vi "Step 7.vi"(8 "error in (no error)":errorcluster, 10 "Water Heater Type":T1, 11 "HeatUp Data in":string[][](array[string])) -> (0 "error out":errorcluster, 1 "110-130 Array":dbl[][](array[numeric]), 2 "Total Energy Expended (W-hr)":dbl, 3 "HP Recovery Time":dbl format="%#.4g", 4 "Watt Hours":cluster{"DBL":dbl[], "DBL":dbl[]}(graph), 5 "TC Avg":cluster{"DBL":dbl[], "DBL":dbl[]}(graph))   [LabVIEW 2016]
uses:
  Type Definitions/HEWH_Type.ctl
  Utility/Custom Pallet Controls/Custom Pallet String.ctl
  <vilib>/Utility/error.llb/DialogType.ctl
panel:
  out "Raw Data":string[][](array[string])
  # "Data with Stripped Header"
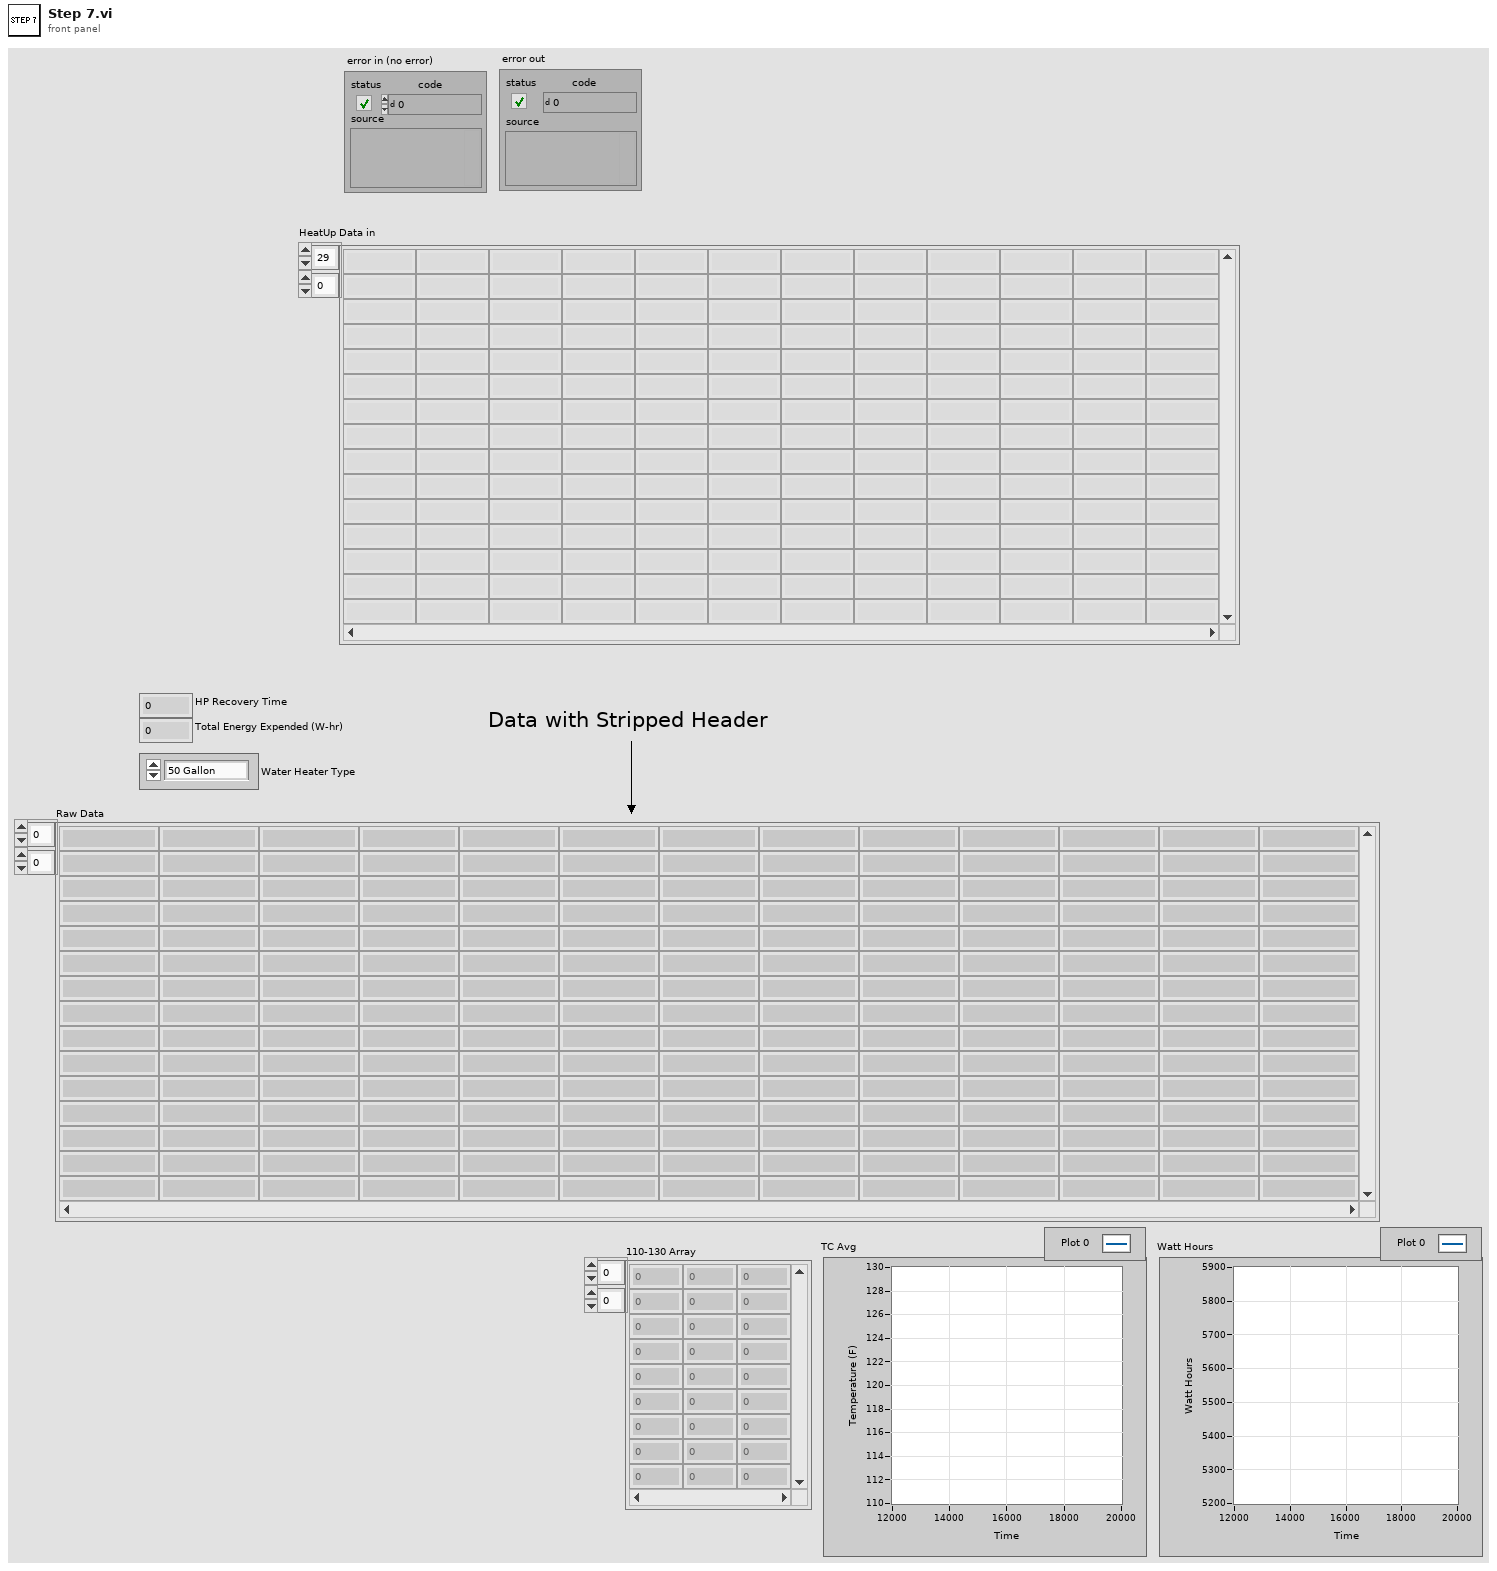
[diagram p1: front panel]
types:
  T1 = typedef "HEWH_Type.ctl" = enum16{"50 Gallon", "80 Gallon"}
  T2 = typedef "Custom Pallet String.ctl" = string
  T3 = cluster{"110-130 Array":dbl[], "110-130 Array":dbl[]}
  T4 = typedef "DialogType.ctl" = u16
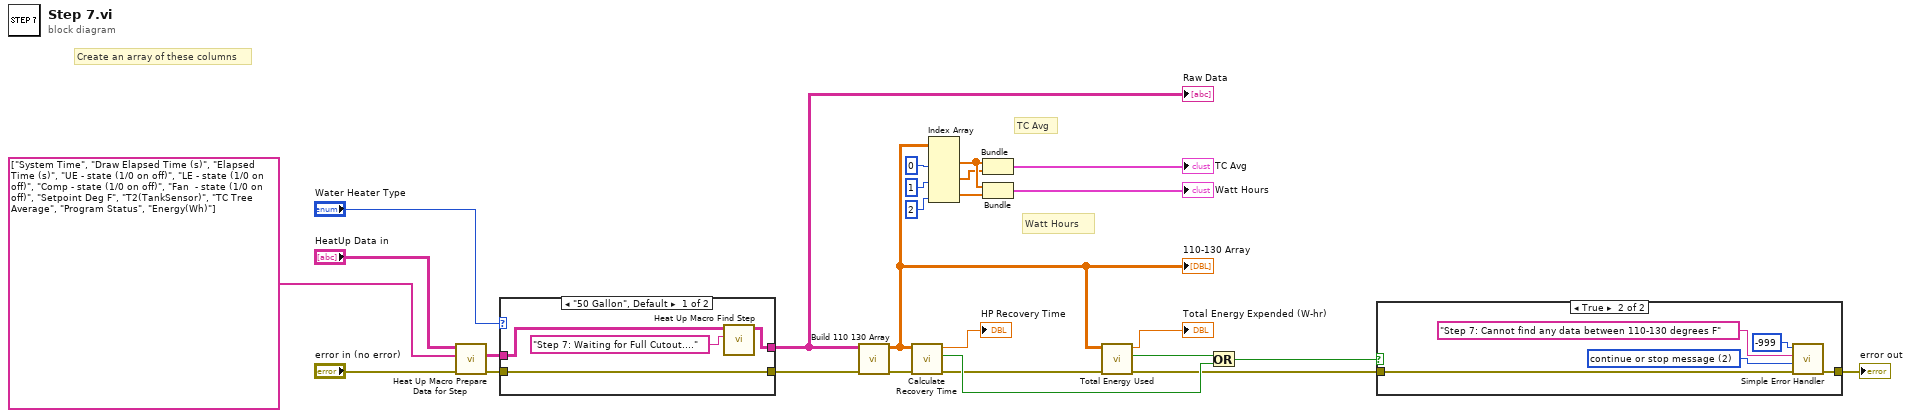
[diagram p0: block diagram]
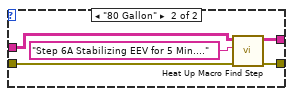
[diagram p2: hidden frame]
diagram:
  # "Watt Hours"
  # "TC Avg"
  # "Create an array of these columns"
  n1 = call "Heat Up Macro Prepare Data for Step.vi"("Error In"="error in (no error)", "Columns Too Search For"=string[] ["System Time", "Draw Elapsed Time (s)", "Elapsed Time (s)", "UE - state (1/0 on off)", "LE - state (1/0 on off)", "Comp - state (1/0 on off)", "Fan  - state (1/0 on off)", "Setpoint Deg F", "T2(TankSensor)", "TC Tree Average", "Program Status", "Energy(Wh)"], "HeatUp Raw Data Input"="HeatUp Data in") -> ("Error Out"=w6:errorcluster, "Heat Up Data with Only Selected Columns"=w9:string[][])  [unwired: 7 in]
  n2 = case shown="\"50 Gallon\", Default" "Water Heater Type" {
    tunnel: w9 -> [w30 w35]
    tunnel: [w28 w33] -> w8
    tunnel: w6 -> [w27 w32]
    tunnel: [w27 w31] -> w5
    frame "50 Gallon", Default {
      n3 = call "Heat Up Macro Find Step.vi"("Search For Step Name"=T2 "Step 7: Waiting for Full Cutout...." ("Message"), "Heat Up Data with Only Selected Columns"=w30) -> ("Filtered Array"=w28:string[][])  [unwired: 7 in, 2 out]
    }
    frame "80 Gallon" {
      n4 = call "Heat Up Macro Find Step.vi"("Error In"=w32, "Search For Step Name"="Step 6A Stabilizing EEV for 5 Min...." ("y"), "Heat Up Data with Only Selected Columns"=w35) -> ("Error Out"=w31:errorcluster, "Filtered Array"=w33:string[][])  [unwired: 6 in, 1 out]
    }
  }
  "Raw Data" <- w8
  n5 = call "Build 110 130 Array.vi"("Error In"=w5, "Filtered Array"=w8) -> ("Error Out"=w3:errorcluster, "110-130 Array"=w20:dbl[][])  [unwired: 8 in]
  "110-130 Array" <- w20
  n6 = call "Calculate Recovery Time.vi"("Error In"=w3, "110-130 Array"=w20) -> ("Error Out"=w2:errorcluster, "No Data Found Between 110-130"=w26:bool, "HP Recovery Time"=→"HP Recovery Time":dbl)  [unwired: 7 in]
  n7 = Index Array(array=w20, index (col) #1=0 ("disabled index (col)"), index (col) #2=1 ("index (col)"), index (col) #3=2 ("index (col)")) -> (element #1=w16:dbl[], element #2=w15:dbl[], element #3=w14:dbl[])  [unwired: 3 in]
  n8 = Bundle("110-130 Array"=w16, "110-130 Array"=w15) -> (→"TC Avg":T3)  [unwired: 1 in]
  n9 = Bundle("110-130 Array"=w16, "110-130 Array"=w14) -> (→"Watt Hours":T3)  [unwired: 1 in]
  n10 = call "Total Energy Used.vi"("Error In"=w2, "110-130 Array"=w20) -> ("Error Out"=w1:errorcluster, "No Data Found Between 110-130"=w25:bool, "Total Energy Expended (W-hr)"=→"Total Energy Expended (W-hr)":dbl)  [unwired: 7 in]
  n11 = Or(x=w25, y=w26) -> (x .or. y?=w23:bool)
  n12 = case shown="True" w23 {
    tunnel: w1 -> [w36 w41]
    tunnel: [w36 w40] -> w24
    frame False {
    }
    frame True {
      w39 = T4 2 items=["no dialog", "OK message", "continue or stop message", "OK message + warnings", "continue/stop + warnings"] ("type of dialog (OK msg:1)")
      n13 = call <vilib>:"Simple Error Handler.vi"("error code (no error:0)"=-999, "error source (\" \")"="Step 7: Cannot find any data between 110-130 degrees F" ("error source (\" \")"), "type of dialog (OK msg:1)"=w39, "error in (no error)"=w41) -> ("error out"=w40:errorcluster)  [unwired: 1 in, 4 out]
    }
  }
  "error out" <- w24
